vi "Resub from string.vi"() -> ()   [LabVIEW 2010]
panel:
  in  "Append":string="_DOS"
  in  "New DIrectory":path
  in  "String":string
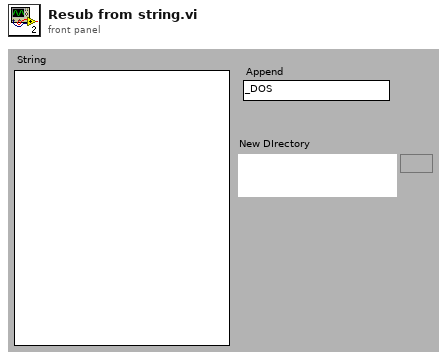
[diagram p1: front panel]
types:
  T1 = cluster{"Command":string, "Value":string, "Comment":string}[]
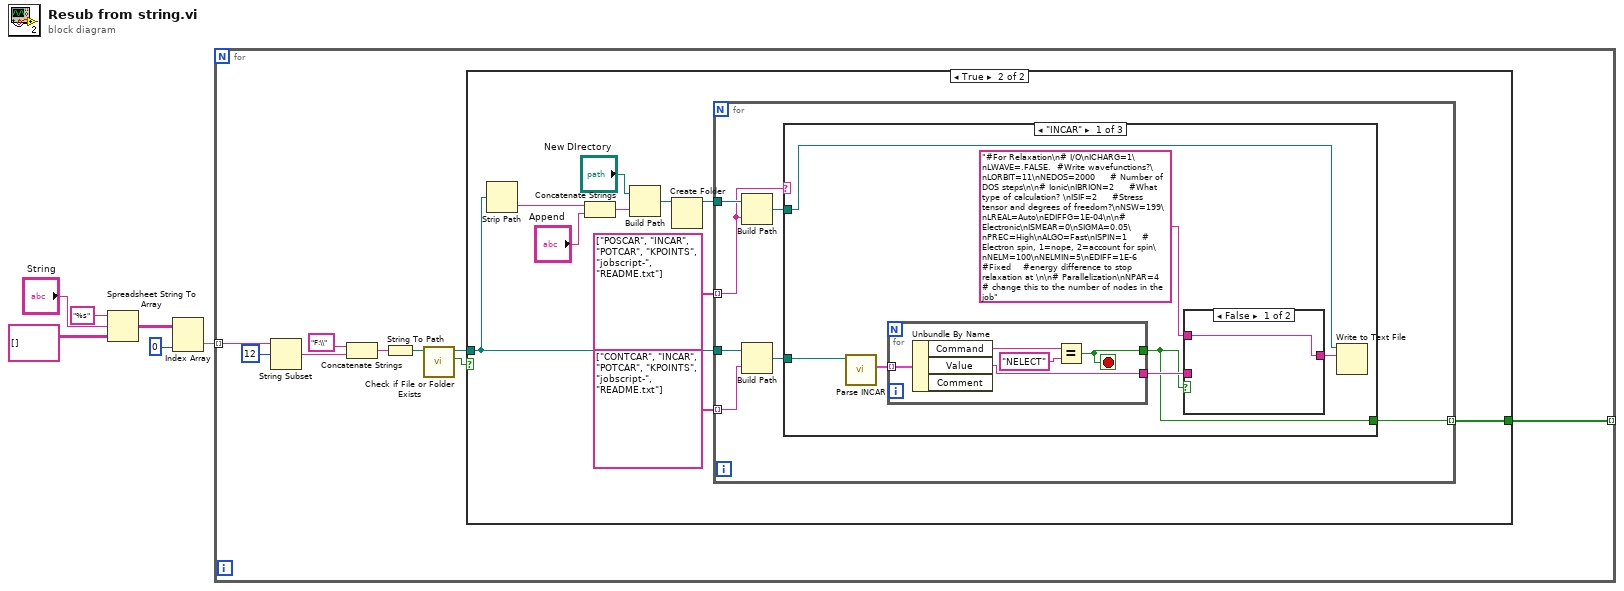
[diagram p0: block diagram]
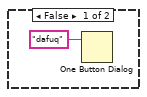
[diagram p2: hidden frame]
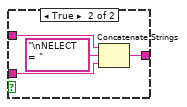
[diagram p3: hidden frame]
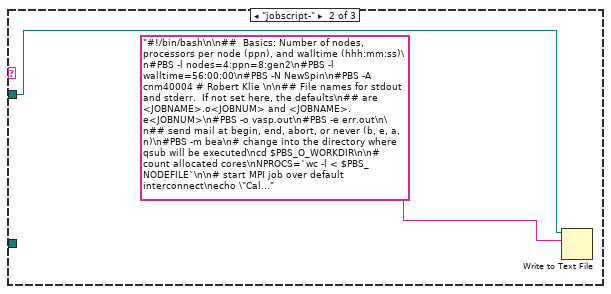
[diagram p4: hidden frame]
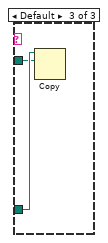
[diagram p5: hidden frame]
diagram:
  n1 = Spreadsheet String To Array(format string="%s", spreadsheet string="String", array type (2D Dbl)=string[][] []) -> (array=w3:string[][])  [unwired: 1 in]
  n2 = Index Array(array=w3, index (col)=0 ("disabled index (col)")) -> (element=w1:string[])  [unwired: 1 in]
  n3 = for {
    tunnel: w1 -> [w15] mode=indexing
    tunnel: [w7] -> _ mode=indexing
    n4 = String Subset(string=w15, offset (0)=12) -> (substring=w13:string)  [unwired: 1 in]
    n5 = Concatenate Strings("F:\\" ("string"), w13) -> (w11:string)
    n6 = String To Path(string=w11) -> (path=w10:path)
    n7 = call <vilib>:"Check if File or Folder Exists.vi"("path"=w10) -> ("file or folder exists?"=w9:bool, "dup path"=w8:path)  [unwired: 8 in, 1 out]
    n8 = case shown="True" w9 {
      tunnel: w8 -> [_ w19]
      tunnel: [_ w17] -> w7
      frame False {
        n9 = One Button Dialog(message="dafuq") -> ()  [unwired: 1 in, 1 out]
      }
      frame True {
        n10 = Strip Path(path=w19) -> (name=w18:string)  [unwired: 1 out]
        n11 = Concatenate Strings(w18, "Append") -> (w20:string)
        n12 = Build Path(base path="New DIrectory", name or relative path=w20) -> (appended path=w25:path)
        n13 = Create Folder(path (use dialog)=w25) -> (created path=w24:path)  [unwired: 2 in, 2 out]
        n14 = for {
          tunnel: w19 -> [w33]
          tunnel: w24 -> [w30]
          tunnel: string[] ["CONTCAR", "INCAR", "POTCAR", "KPOINTS", "jobscript-", "README.txt"] -> [w32] mode=indexing
          tunnel: string[] ["POSCAR", "INCAR", "POTCAR", "KPOINTS", "jobscript-", "README.txt"] -> [w28] mode=indexing
          tunnel: [w27] -> w17 mode=indexing
          n15 = Build Path(base path=w30, name or relative path=w28) -> (appended path=w29:path)
          n16 = Build Path(base path=w33, name or relative path=w32) -> (appended path=w31:path)
          n17 = case shown="\"INCAR\"" w28 {
            tunnel: w31 -> [w35 _ w54]
            tunnel: w29 -> [w40 w52 w53]
            tunnel: [w34 _ _] -> w27
            frame "INCAR" {
              n18 = call "Parse INCAR.vi"("INCAR File"=w35) -> ("INCAR Raw Commands"=w39:T1)  [unwired: 6 in, 4 out]
              n19 = for {
                tunnel: w39 -> [w50] mode=indexing
                tunnel: [w47] -> w37
                tunnel: [w46] -> w34
                stop <- w46 stop-if-true
                n20 = Unbundle By Name(w50) -> ("Command"=w49:string, "Value"=w47:string)  [unwired: 1 out]
                n21 = Equal?(x=w49, y="NELECT") -> (x = y?=w46:bool)
              }
              n22 = case shown="False" w34 {
                tunnel: "#For Relaxation\n# I/O\nICHARG=1\nLWAVE=.FALSE.  #Write wavefunctions?\nLORBIT=11\nNEDOS=2000     # Number of DOS steps\n\n# Ionic\nIBRION=2     #What type of calculation? \nISIF=2     #Stress tensor and degrees of freedom?\nNSW=199\nLREAL=Auto\nEDIFFG=1E-04\n\n# Electronic\nISMEAR=0\nSIGMA=0.05\nPREC=High\nALGO=Fast\nISPIN=1     # Electron spin, 1=nope, 2=account for spin\nNELM=100\nNELMIN=5\nEDIFF=1E-6  #Fixed    #energy difference to stop relaxation at \n\n# Parallelization\nNPAR=4     # change this to the number of nodes in the job" ("text") -> [w41 w45]
                tunnel: w37 -> [_ w43]
                tunnel: [w41 w42] -> w36
                frame False {
                }
                frame True {
                  n23 = Concatenate Strings(w45, "\nNELECT = " ("string"), w43) -> (w42:string)
                }
              }
              n24 = Write to Text File(file (use dialog)=w40, text=w36) -> ()  [unwired: 2 in, 3 out]
            }
            frame "jobscript-" {
              n25 = Write to Text File(file (use dialog)=w52, text="#!/bin/bash\n\n##  Basics: Number of nodes, processors per node (ppn), and walltime (hhh:mm:ss)\n#PBS -l nodes=4:ppn=8:gen2\n#PBS -l walltime=56:00:00\n#PBS -N NewSpin\n#PBS -A cnm40004 # Robert Klie \n\n## File names for stdout and stderr.  If not set here, the defaults\n## are <JOBNAME>.o<JOBNUM> and <JOBNAME>.e<JOBNUM>\n#PBS -o vasp.out\n#PBS -e err.out\n\n## send mail at begin, end, abort, or never (b, e, a, n)\n#PBS -m bea\n# change into the directory where qsub will be executed\ncd $PBS_O_WORKDIR\n\n# count allocated cores\nNPROCS=`wc -l < $PBS_NODEFILE`\n\n# start MPI job over default interconnect\necho \"Calc Incomplete\" > IncompleteCalc\nmpirun -machinefile $PBS_NODEFILE -np $NPROCS vasp\nrm CHG\nrm IncompleteCalc") -> ()  [unwired: 2 in, 3 out]
            }
            frame Default {
              n26 = Copy(10:w53, 11:w54) -> ()  [unwired: 3 in, 3 out]
            }
          }
        }
      }
    }
  }
